vi "Func_AddToLibrary.vi"(8 "error in (no error)":errorcluster, 10 "Library Path":path, 11 "VI Path":path) -> (0 "error out":errorcluster)   [LabVIEW 2010, in "TemplateGenerator.lvlib"]
uses:
  TemplateGenerator.lvlib
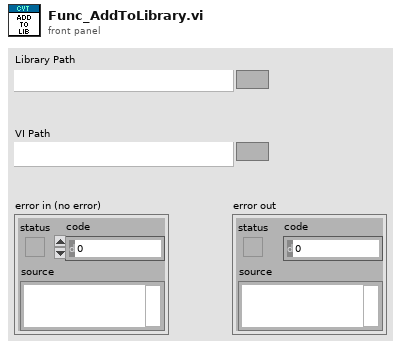
[diagram p1: front panel]
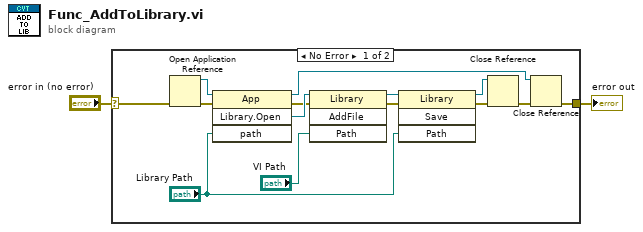
[diagram p0: block diagram]
diagram:
  n1 = case shown="No Error" "error in (no error)" {
    selector: "error in (no error)" -> [w3 w17]
    tunnel: [w6 w17] -> w2
    frame No Error {
      n2 = Open Application Reference(8:w3) -> (0:w15:errorcluster, 3:w16:refnum<vi>)  [unwired: 3 in]
      n3 = invoke class="App" method="Library.Open"(reference=w16, error in=w15, "path"="Library Path") -> (reference out=w7:refnum<vi>, error out=w4:errorcluster, "Open Library"=w14:refnum<vi>)  [unwired: 1 in, 1 out]
      n4 = invoke class="Library" method="AddFile"(reference=w14, error in=w4, "Path"="VI Path") -> (reference out=w13:refnum<vi>, error out=w12:errorcluster)  [unwired: 1 in, 2 out]
      n5 = invoke class="Library" method="Save"(reference=w13, error in=w12, "Path"="Library Path") -> (reference out=w10:refnum<vi>, error out=w9:errorcluster)  [unwired: 1 in, 2 out]
      n6 = Close Reference(reference=w10, error in (no error)=w9) -> (error out=w8:errorcluster)
      n7 = Close Reference(reference=w7, error in (no error)=w8) -> (error out=w6:errorcluster)
    }
    frame Error {
    }
  }
  "error out" <- w2
